vi "Calculate position from parameters.vi"(6 "Current step":dbl, 8 "error in (no error)":errorcluster, 9 "mm/step":dbl, 10 "Tipo de paso":u8(ring)=1 items=["", "Medio paso", "Paso completo"], 11 "Motor direction":u8) -> (0 "error out":errorcluster, 3 "Position adjustment":dbl)   [LabVIEW 2020, in "Control de MaP.lvlib"]
doc: "Converts the number of steps to mm. The VI takes into account the direction of movement and the type of step. Currently support only full and half stepping."
uses:
  Control de MaP.lvlib
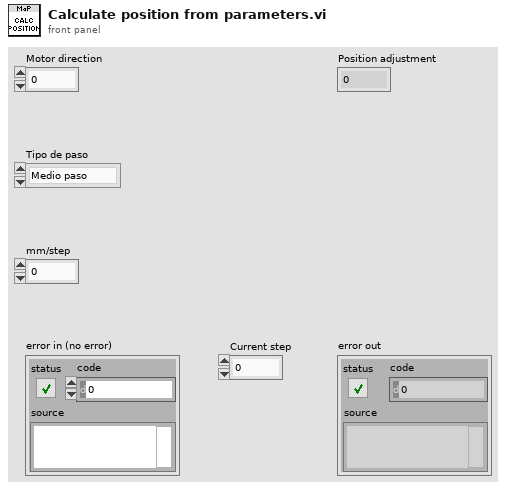
[diagram p1: front panel]
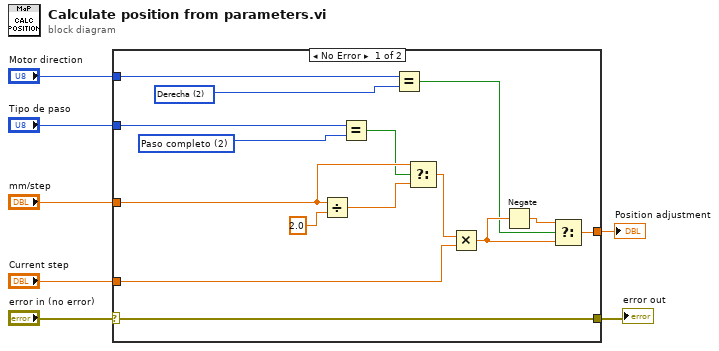
[diagram p0: block diagram]
diagram:
  n1 = case shown="No Error" "error in (no error)" {
    selector: "error in (no error)" -> [w10 w23]
    tunnel: "mm/step" -> [w20 _]
    tunnel: [w19 w24] -> w6
    tunnel: "Motor direction" -> [w15 _]
    tunnel: "Tipo de paso" -> [w12 _]
    tunnel: "Current step" -> [w11 w24]
    tunnel: [w10 w23] -> w2
    frame No Error {
      w8 = u8 2 items=["", "Medio paso", "Paso completo"] ("Tipo de paso")
      w9 = u8 2 items=["", "Izquierda", "Derecha"] ("Dirección")
      n2 = Divide(x=w20, y=2.0) -> (x/y=w22:dbl)
      n3 = Equal?(x=w12, y=w8) -> (x = y?=w13:bool)
      n4 = Equal?(x=w15, y=w9) -> (x = y?=w16:bool)
      n5 = Select(t=w20, s=w13, f=w22) -> (s? t:f=w14:dbl)
      n6 = Multiply(x=w14, y=w11) -> (x*y=w18:dbl)
      n7 = Negate(x=w18) -> (-x=w17:dbl)
      n8 = Select(t=w17, s=w16, f=w18) -> (s? t:f=w19:dbl)
    }
    frame Error {
    }
  }
  "Position adjustment" <- w6
  "error out" <- w2
